vi "探测器列表-重排设备.vi"(5 "元素名[]-探测器信息":string[](array[string]), 7 "table名-探测器列表":string, 8 "error in (no error)":errorcluster, 9 "新顺序":i32[](array[numeric]), 10 "探测器清单":T1[](array[typedef]), 11 "数据库引用":T4) -> (0 "error out":errorcluster, 2 "探测器清单 new":T1[](array[typedef]), 3 "connection reference out":T4)   [LabVIEW 2017]
uses:
  <vilib>/addons/database/Connection.llb/Conn ObjectReference.ctl
  <vilib>/addons/database/NI_Database_API.lvlib
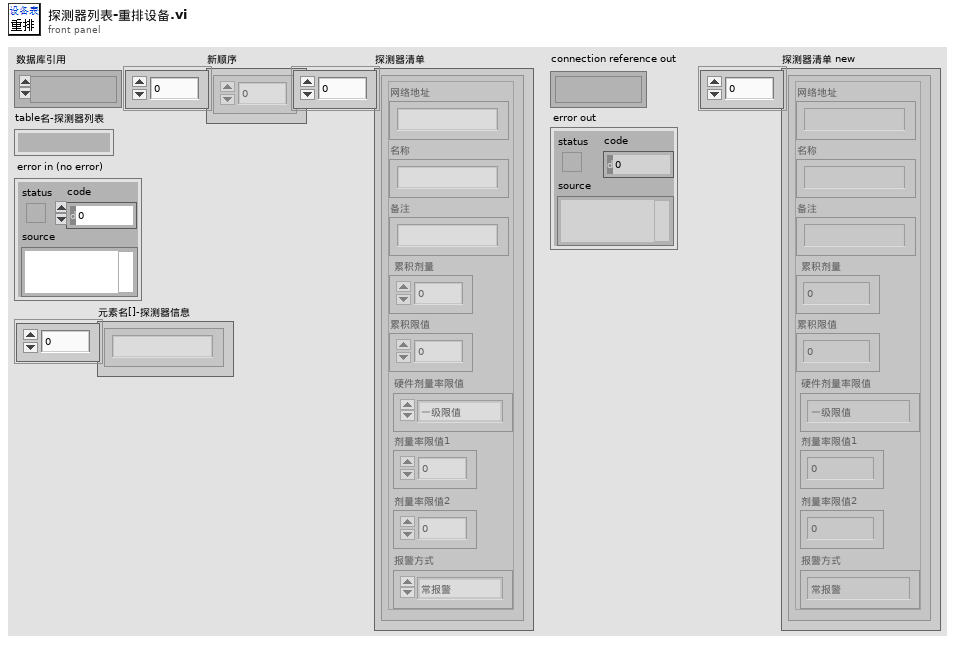
[diagram p1: front panel]
types:
  T1 = typedef "探测器信息.ctl" = cluster{"网络地址":string, "名称":string, "备注":string, "累积剂量":dbl, "累积限值":dbl, "硬件剂量率限值":T2, "剂量率限值1":dbl, "剂量率限值2":dbl, "报警方式":T3}
  T2 = typedef "探头剂量率限值选择.ctl" = enum16{"一级限值", "二级限值"}
  T3 = typedef "报警方式选择.ctl" = enum16{"常报警", "自动静音", "手动静音"}
  T4 = typedef "NI_Database_API.lvlib/Conn ObjectReference.ctl" = refnum<k1>
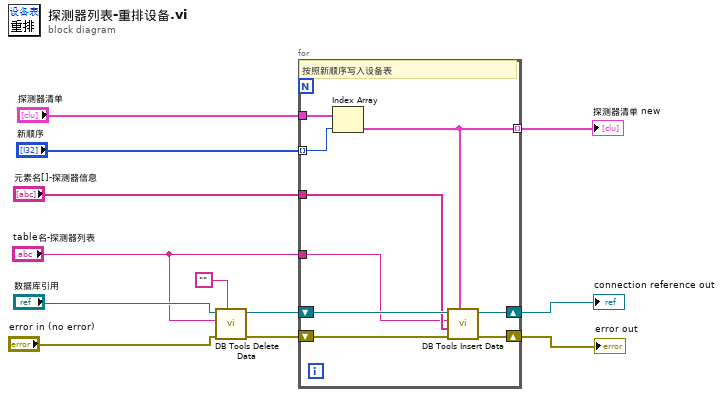
[diagram p0: block diagram]
diagram:
  n1 = call <vilib>:"DB Tools Delete Data.vi"("condition"="", "error in (no error)"="error in (no error)", "table"="table名-探测器列表", "connection reference"="数据库引用") -> ("error out"=w6:errorcluster, "connection reference out"=w7:T4)  [unwired: 6 in]
  n2 = for {
    tunnel: "探测器清单" -> [w21]
    tunnel: "新顺序" -> [w20] mode=indexing
    shift-right: [w16] -> w3
    shift-left: w7 -> [w19]
    shift-right: [w17] -> w2
    shift-left: w6 -> [w18]
    tunnel: "元素名[]-探测器信息" -> [w15]
    tunnel: [w14] -> w4 mode=indexing
    tunnel: "table名-探测器列表" -> [w13]
    # "按照新顺序写入设备表"
    n3 = Index Array(array=w21, index=w20) -> (element=w14:T1)
    n4 = call <vilib>:"DB Tools Insert Data.vi"("data"=w14, "error in (no error)"=w18, "columns"=w15, "table"=w13, "connection reference"=w19) -> ("error out"=w17:errorcluster, "connection reference out"=w16:T4)  [unwired: 5 in]
  }
  "connection reference out" <- w3
  "error out" <- w2
  "探测器清单 new" <- w4
